vi "komendyGeneratora.vi"(8 "Akcja":T5, 11 "Generator_ZKP_Wejście":T1={"Parametry sygnału"={"amplitude"=1.0, "chirp duration [s]"=4.0, "frequency range"={"start frequency [Hz]"=20.0, "stop frequency [Hz]"=20000.0}}, "Rodzaj sygnału"=enum."pink noise", "command"=enum."play"}) -> (3 "Generator_ZKP_Wyjście":T1={"Parametry sygnału"={"amplitude"=1.0, "chirp duration [s]"=4.0, "frequency range"={"start frequency [Hz]"=20.0, "stop frequency [Hz]"=20000.0}}, "Rodzaj sygnału"=enum."pink noise", "command"=enum."play"})   [LabVIEW 2014]
uses:
  Generator_ZKP_Parametry.ctl
  signal parameters.ctl
  signal type.ctl
  command.ctl
  glownaMaszynaStanowVIs/AkcjaGFV.ctl
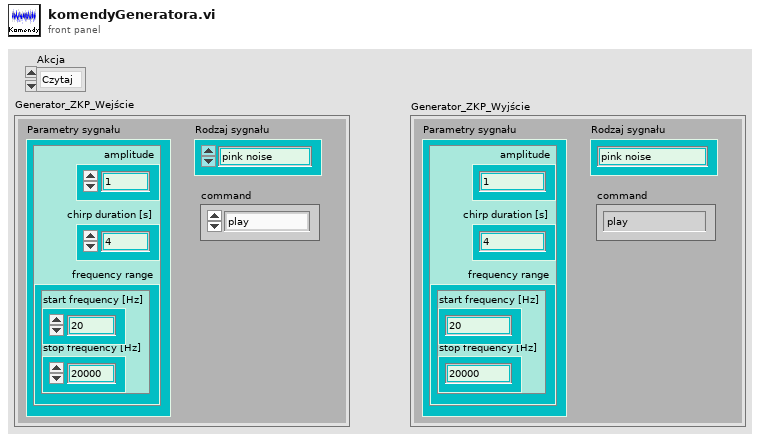
[diagram p1: front panel]
types:
  T1 = typedef "Generator_ZKP_Parametry.ctl" = cluster{"Parametry sygnału":T2, "Rodzaj sygnału":T3, "command":T4}
  T2 = typedef "signal parameters.ctl" = cluster{"amplitude":dbl, "chirp duration [s]":dbl, "frequency range":cluster{"start frequency [Hz]":dbl, "stop frequency [Hz]":dbl}}
  T3 = typedef "signal type.ctl" = enum16{"pink noise", "white noise", "chirp"}
  T4 = typedef "command.ctl" = enum16{"play", "stop", "exit"}
  T5 = typedef "AkcjaGFV.ctl" = enum16{"Czytaj", "Zapisz", "Reset"}
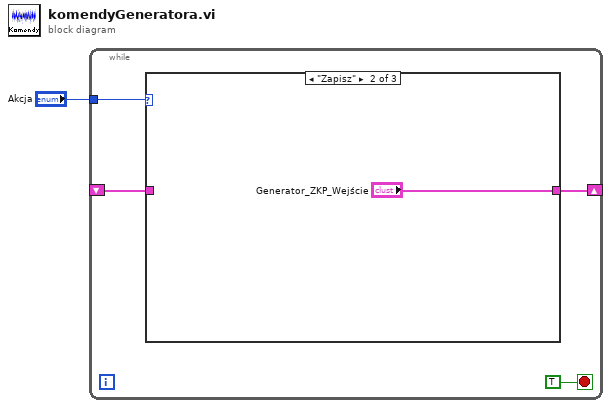
[diagram p0: block diagram]
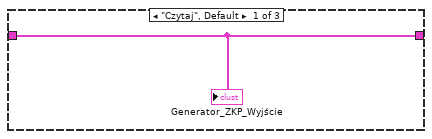
[diagram p2: hidden frame]
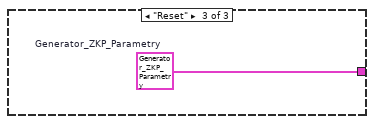
[diagram p3: hidden frame]
diagram:
  n1 = while {
    tunnel: "Akcja" -> [w5]
    shift-right: [w4] -> _
    shift-left: _ -> [w3]
    stop <- TRUE stop-if-true
    n2 = case shown="\"Zapisz\"" w5 {
      tunnel: [w6 "Generator_ZKP_Wejście" w8] -> w4
      tunnel: w3 -> [w6 _ _]
      frame "Czytaj", Default {
        "Generator_ZKP_Wyjście" <- w6
      }
      frame "Zapisz" {
      }
      frame "Reset" {
        w8 = T1 {"Parametry sygnału"={"amplitude"=1.0, "chirp duration [s]"=4.0, "frequency range"={"start frequency [Hz]"=20.0, "stop frequency [Hz]"=20000.0}}, "Rodzaj sygnału"=enum."pink noise", "command"=enum."play"}  # Generator_ZKP_Parametry
      }
    }
  }
